vi "User Input Que Parser (SubVI).vi"(4 "DATA IN":dbl[](array[numeric])) -> (0 "Valve States":dbl[](array[numeric]), 1 "Bang":dbl[](array[numeric]), 2 "Sequences":dbl[](array[numeric]), 3 "Timer":dbl[](array[numeric]), 5 "Abort State":dbl[](array[numeric]), 6 "GO States":dbl[](array[numeric]), 7 "Blank":dbl[](array[numeric]), 8 "Phase":dbl[](array[numeric]))   [LabVIEW 2020]
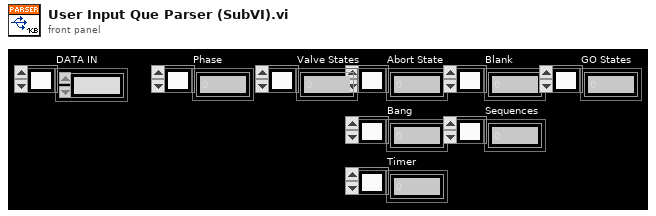
[diagram p1: front panel]
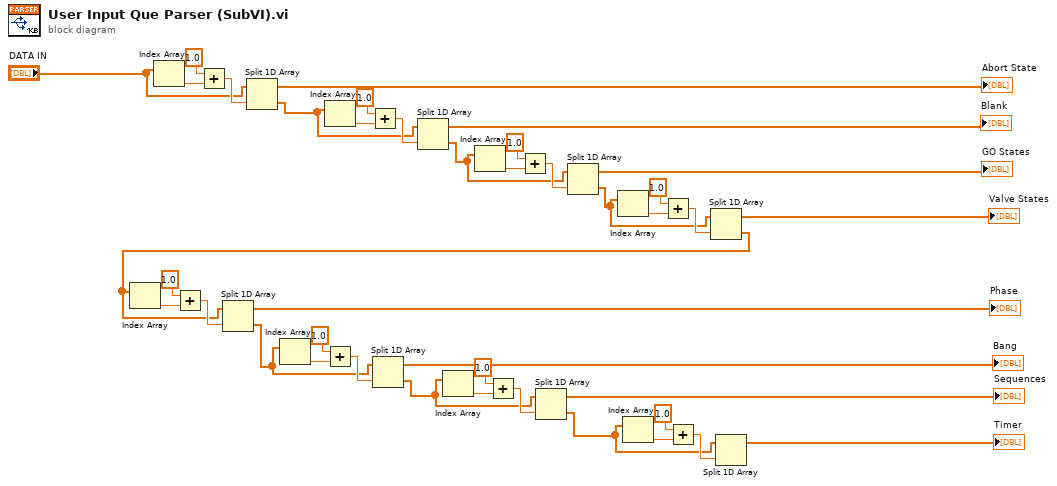
[diagram p0: block diagram]
diagram:
  n1 = Index Array(array="DATA IN") -> (element=w38:dbl)  [unwired: 1 in]
  n2 = Add(x=1.0, y=w38) -> (x+y=w39:dbl)
  n3 = Split 1D Array(array="DATA IN", index=w39) -> (first subarray=→"Abort State":dbl[], second subarray=w21:dbl[])
  n4 = Index Array(array=w21) -> (element=w37:dbl)  [unwired: 1 in]
  n5 = Add(x=1.0, y=w37) -> (x+y=w36:dbl)
  n6 = Split 1D Array(array=w21, index=w36) -> (first subarray=→"Blank":dbl[], second subarray=w20:dbl[])
  n7 = Index Array(array=w20) -> (element=w33:dbl)  [unwired: 1 in]
  n8 = Add(x=1.0, y=w33) -> (x+y=w32:dbl)
  n9 = Split 1D Array(array=w20, index=w32) -> (first subarray=→"GO States":dbl[], second subarray=w19:dbl[])
  n10 = Index Array(array=w19) -> (element=w30:dbl)  [unwired: 1 in]
  n11 = Add(x=1.0, y=w30) -> (x+y=w29:dbl)
  n12 = Split 1D Array(array=w19, index=w29) -> (first subarray=→"Valve States":dbl[], second subarray=w9:dbl[])
  n13 = Index Array(array=w9) -> (element=w27:dbl)  [unwired: 1 in]
  n14 = Add(x=1.0, y=w27) -> (x+y=w26:dbl)
  n15 = Split 1D Array(array=w9, index=w26) -> (first subarray=→"Phase":dbl[], second subarray=w18:dbl[])
  n16 = Index Array(array=w18) -> (element=w24:dbl)  [unwired: 1 in]
  n17 = Add(x=1.0, y=w24) -> (x+y=w23:dbl)
  n18 = Split 1D Array(array=w18, index=w23) -> (first subarray=→"Bang":dbl[], second subarray=w10:dbl[])
  n19 = Index Array(array=w10) -> (element=w17:dbl)  [unwired: 1 in]
  n20 = Add(x=1.0, y=w17) -> (x+y=w16:dbl)
  n21 = Split 1D Array(array=w10, index=w16) -> (first subarray=→"Sequences":dbl[], second subarray=w11:dbl[])
  n22 = Index Array(array=w11) -> (element=w14:dbl)  [unwired: 1 in]
  n23 = Add(x=1.0, y=w14) -> (x+y=w13:dbl)
  n24 = Split 1D Array(array=w11, index=w13) -> (first subarray=→"Timer":dbl[])  [unwired: 1 out]
